vi "readDataArray.vi"(8 "error in (no error)":errorcluster, 10 "array":string[][](array[string]), 11 "K2602FileReader in":refnum<class "K2602FileReader.lvclass">) -> (0 "error out":errorcluster, 3 "K2602FileReader out":refnum<class "K2602FileReader.lvclass">)   [LabVIEW 2011, in "Tools.lvlib" / "Filing.lvlib" / "K2602FileReader.lvclass"]
uses:
  K2602FileReader.lvclass
  K2602FileReader.lvclass/K2602FileReader.ctl
  Hal/Channels/VoltOutput/AnalogOutput.lvclass
panel:
  out "times":dbl[](array[numeric]) format="%#_6f"
  out "data":dbl[][](array[numeric])
  out "Defaults":dbl[](array[numeric])
  out "channelAddresses":string[](array[string])
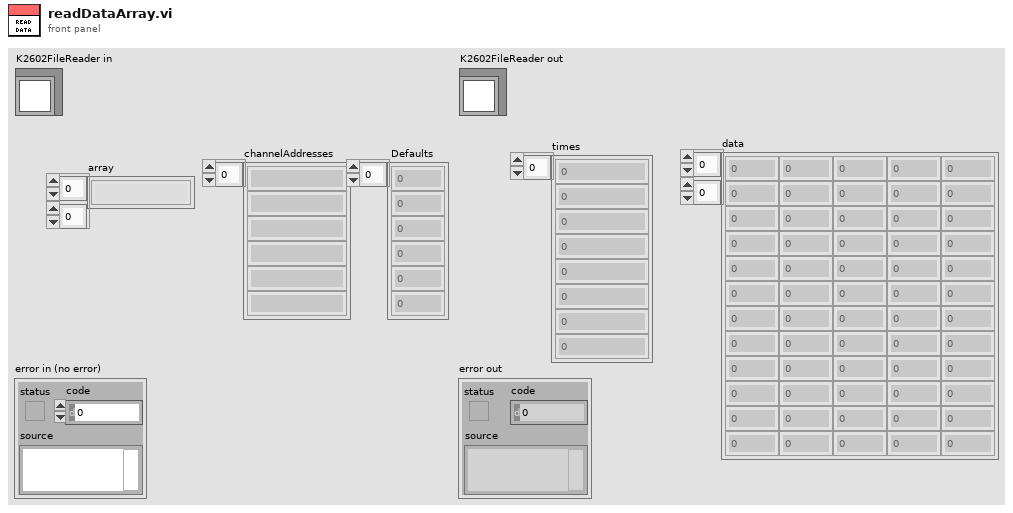
[diagram p1: front panel]
types:
  T1 = cluster{"Clock source":string, "Clock rate":dbl, "Start trigger line":string, "Sample Rate":dbl, "Sample No.":dbl}
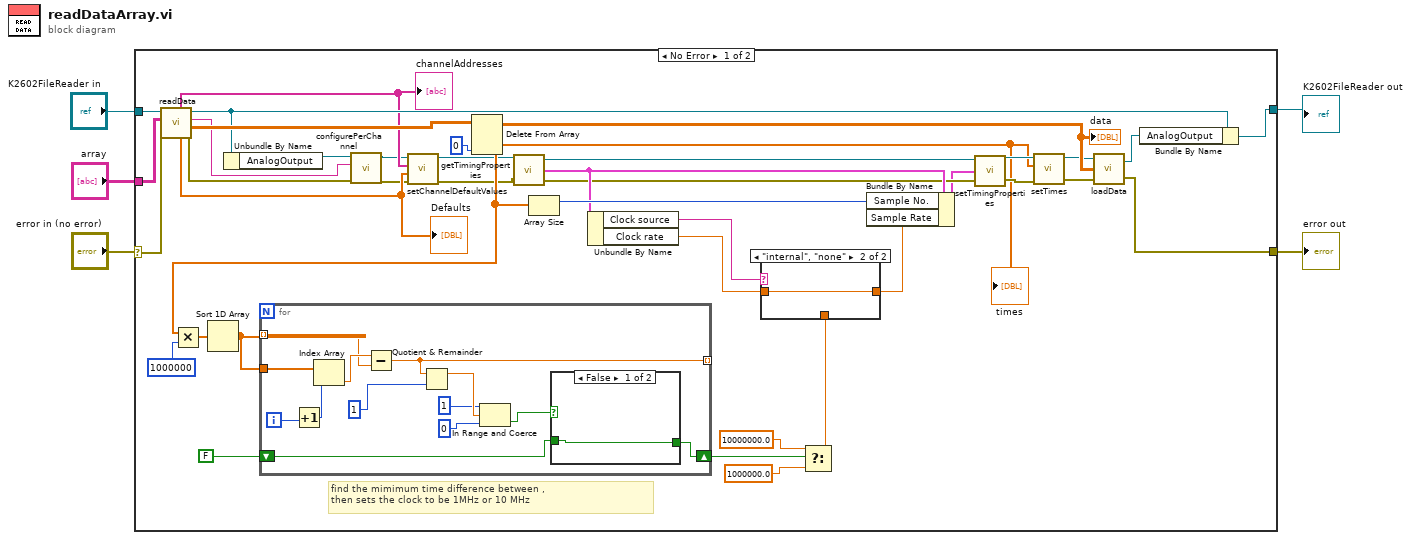
[diagram p0: block diagram]
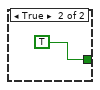
[diagram p3: hidden frame]
diagram:
  n1 = case shown="No Error" "error in (no error)" {
    selector: "error in (no error)" -> [w43 w63]
    tunnel: "K2602FileReader in" -> [w45 w64]
    tunnel: "array" -> [w44 _]
    tunnel: [w16 w64] -> w2
    tunnel: [w19 w63] -> w1
    frame No Error {
      # "find the mimimum time difference between ,\nthen sets the clock to be 1MHz or 10 MHz"
      n2 = call-dynamic "readData.vi"("error in (no error)"=w43, "array"=w44, "FileReader in"=w45) -> ("error out"=w6:errorcluster, "Array"=w26:dbl[][], "channels"=w7:string, "FileReader out"=w18:refnum<class "K2602FileReader.lvclass">, "Defaults"=w11:dbl[], "channelAddresses"=w12:string[])  [unwired: 3 in]
      "Defaults" <- w11
      "channelAddresses" <- w12
      n3 = Unbundle By Name(w18) -> ("AnalogOutput"=w8:refnum<class "AnalogOutput.lvclass">)
      n4 = call-dynamic "configurePerChannel.vi"("error in (no error)"=w6, "physical channels"=w7, "AnalogOutput in"=w8) -> ("error out"=w9:errorcluster, "AnalogOutput out"=w10:refnum<class "AnalogOutput.lvclass">)  [unwired: 7 in]
      n5 = call "setChannelDefaultValues.vi"("error in (no error)"=w9, "calibratedValues"=w11, "channel_addresses"=w12, "AnalogOutput in"=w10) -> ("error out"=w14:errorcluster, "AnalogOutput out"=w13:refnum<class "AnalogOutput.lvclass">)  [unwired: 6 in]
      n6 = Delete From Array(array=w26, index (col)=0 ("disabled index (col)")) -> (deleted portion=w15:dbl[], array with subset deleted=w24:dbl[][])  [unwired: 2 in]
      "data" <- w24
      "times" <- w15
      n7 = Multiply(x=w15, y=1000000) -> (x*y=w36:dbl[])
      n8 = Sort 1D Array(array=w36) -> (sorted array=w41:dbl[])
      n9 = for {
        tunnel: w41 -> [w56] mode=indexing
        tunnel: w41 -> [w60]
        tunnel: [w51] -> _ mode=indexing
        shift-right: [w48] -> w39
        shift-left: FALSE -> [w49]
        i -> [w59]
        n10 = Increment(x=w59) -> (x+1=w58:i32)
        n11 = Index Array(array=w60, index=w58) -> (element=w57:dbl)
        n12 = Subtract(x=w57, y=w56) -> (x-y=w51:dbl)
        n13 = Quotient & Remainder(x=w51, y=1) -> (x-y*floor(x/y)=w54:dbl)  [unwired: 1 out]
        n14 = In Range and Coerce(upper limit=1, x=w54, lower limit=0) -> (In Range?=w50:bool)  [unwired: 1 out]
        n15 = case shown="False" w50 {
          tunnel: w49 -> [w61 _]
          tunnel: [w61 TRUE] -> w48
          frame False {
          }
          frame True {
          }
        }
      }
      n16 = call "getTimingProperties.vi"("AnalogOutput.lvclass in"=w13, "error in (no error)"=w14) -> ("AnalogOutput.lvclass out"=w29:refnum<class "AnalogOutput.lvclass">, "Timing"=w34:T1, "error out"=w28:errorcluster)
      n17 = Array Size(array=w15) -> (size(s)=w42:i32)
      n18 = Unbundle By Name(w34) -> ("Clock source"=w33:string, "Clock rate"=w31:dbl)
      n19 = Select(t=10000000.0, s=w39, f=1000000.0) -> (s? t:f=w32:dbl)
      n20 = case shown="\"internal\", \"none\"" w33 {
        tunnel: w32 -> [w46 _]
        tunnel: w31 -> [_ w47]
        tunnel: [w46 w47] -> w30
        frame Default {
        }
        frame "internal", "none" {
        }
      }
      n21 = Bundle By Name(cluster=w34, "Sample No."=w42, "Sample Rate"=w30) -> (w27:T1)
      n22 = call "setTimingProperties.vi"("error in (no error)"=w28, "Timing"=w27, "AnalogOutput.lvclass in"=w29) -> ("error out"=w21:errorcluster, "AnalogOutput.lvclass out"=w23:refnum<class "AnalogOutput.lvclass">)
      n23 = call "setTimes.vi"("error in (no error)"=w21, "times"=w15, "AnalogOutput in"=w23) -> ("error out"=w20:errorcluster, "AnalogOutput out"=w22:refnum<class "AnalogOutput.lvclass">)  [unwired: 7 in]
      n24 = call-dynamic "loadData.vi"("error in (no error)"=w20, "Data"=w24, "AnalogOutput in"=w22) -> ("error out"=w19:errorcluster, "AnalogOutput out"=w17:refnum<class "AnalogOutput.lvclass">)
      n25 = Bundle By Name(cluster=w18, "AnalogOutput"=w17) -> (w16:refnum<class "K2602FileReader.lvclass">)
    }
    frame Error {
    }
  }
  "error out" <- w1
  "K2602FileReader out" <- w2
